vi "Acquire DI.vi"(8 "error in (no error)":errorcluster, 11 "PXIe 6363 in":refnum<class "PXIe 6363.lvclass">) -> (0 "error out":errorcluster, 2 "Acquire DI":bool[](array[boolean]), 3 "PXIe 6363 out":refnum<class "PXIe 6363.lvclass">)   [LabVIEW 2023, in "DAQ Hardware.lvlib" / "PXIe 6363.lvclass"]
uses:
  PXIe 6363.lvclass
  PXIe 6363.lvclass/PXIe 6363.ctl
  <vilib>/DAQmx/read.llb/DAQmx Read (Digital 1D Bool NChan 1Samp 1Line).vi
  <vilib>/DAQmx/miscellaneous.llb/DAQmx Fill In Error Info.vi
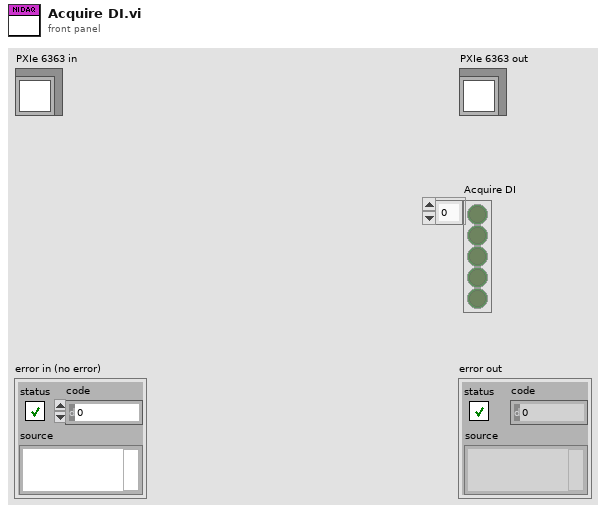
[diagram p1: front panel]
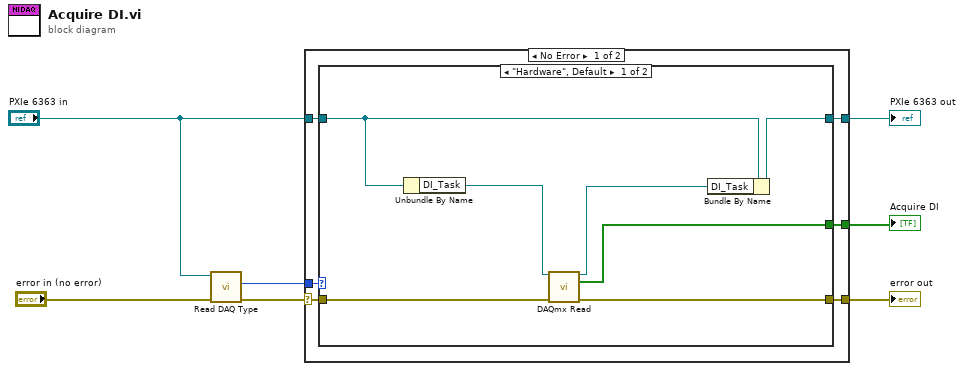
[diagram p0: block diagram]
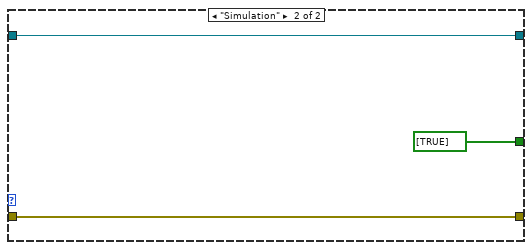
[diagram p2: hidden frame]
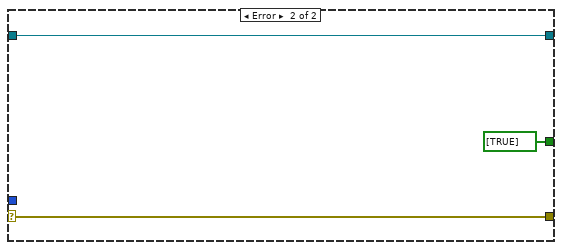
[diagram p3: hidden frame]
diagram:
  n1 = call-dynamic "Read DAQ Type.vi"("error in (no error)"="error in (no error)", "PXIe 6363 in"="PXIe 6363 in") -> ("error out"=w7:errorcluster, "DAQ Type"=w6:enum16{"Hardware", "Simulation"})  [unwired: 7 in, 1 out]
  n2 = case shown="No Error" w7 {
    selector: w7 -> [w11 w24]
    tunnel: w6 -> [w13 _]
    tunnel: "PXIe 6363 in" -> [w12 w26]
    tunnel: [w10 w26] -> w2
    tunnel: [w9 w24] -> w1
    tunnel: [w8 bool[] [TRUE] ("data")] -> w3
    frame No Error {
      n3 = case shown="\"Hardware\", Default" w13 {
        tunnel: w12 -> [w19 w22]
        tunnel: w11 -> [w20 w21]
        tunnel: [w18 w22] -> w10
        tunnel: [w17 w21] -> w9
        tunnel: [w16 bool[] [TRUE] ("data")] -> w8
        frame "Hardware", Default {
          n4 = Unbundle By Name(w19) -> ("DI_Task"=w15:refnum<k21>)
          n5 = call-poly <vilib>:"DAQmx Read.vi"("task/channels in"=w15, "error in"=w20) -> ("task out"=w14:refnum<k21>, "data"=w16:bool[], "error out"=w17:errorcluster)  [unwired: 11 in]
          n6 = Bundle By Name(cluster=w19, "DI_Task"=w14) -> (w18:refnum<class "PXIe 6363.lvclass">)
        }
        frame "Simulation" {
        }
      }
    }
    frame Error {
    }
  }
  "error out" <- w1
  "PXIe 6363 out" <- w2
  "Acquire DI" <- w3
